vi "DEVICE_COUNT.vi"() -> ()   [LabVIEW 2026]
panel:
  in  "Selected device Count":i32
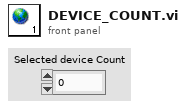
[diagram p1: front panel]
diagram:
